vi "PMX-4EX-SA Command Generator.vi"(0 "COMMAND":T1=enum."getDeviceId", 5 "args":string[](array[string]), 7 "AXIS":u16(ring) items=["X", "Y", "Z", "U"]) -> (6 "COMMAND":string)   [LabVIEW 2018]
doc: "converts a user friendly request to an actual (raw) string command for the Performax API\n\nProduced By:\n\nChristopher Lemieux\nTest and Automation Engineer\ntestengnr@yahoo.com"
uses:
  PerformaxLV_v103.llb/commandsnew.ctl
panel:
  # "LIBRARY FILE ADJUSTED FOR X,Y,Z,U"
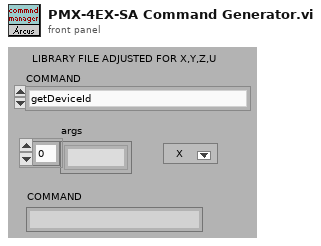
[diagram p1: front panel]
types:
  T1 = typedef "commandsnew.ctl" = enum16{"clearErr", "constJogNeg", "constJogPos", "getAccel", "getDeviceId", "getFirmwareVer", "getHighSpeed", "getIdleAmp", "getLowSpeed", "getMicroStep", "getMotorStatus", "getPolarity", "getPosition", "getProdId", "getPwrStatus", "getRunAmp", "getStatus", "getTemp", "homeNeg", "homePos", "moveToPosition", "powerDown", "powerUp", "setAccel", "setDeviceId", "setHighSpeed", "setIdleAmp", "setLowSpeed", "setMicroStep", "setPolarityLow", "setPolarityHigh", "setPosition", "setRunAmp", "stopFast", "stopSlow"}
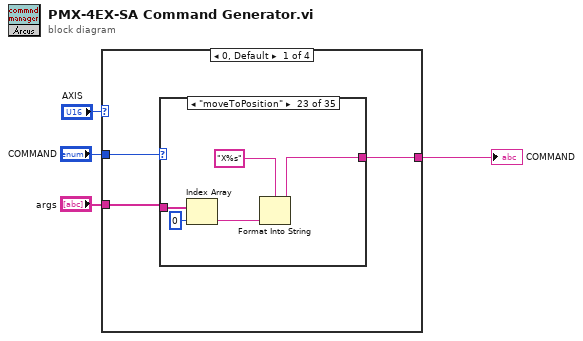
[diagram p0: block diagram]
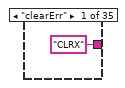
[diagram p2: hidden frame]
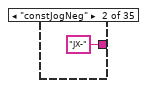
[diagram p3: hidden frame]
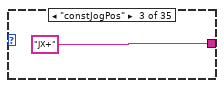
[diagram p4: hidden frame]
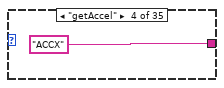
[diagram p5: hidden frame]
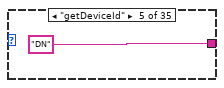
[diagram p6: hidden frame]
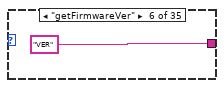
[diagram p7: hidden frame]
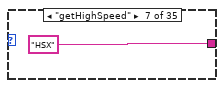
[diagram p8: hidden frame]
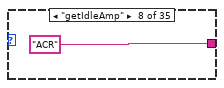
[diagram p9: hidden frame]
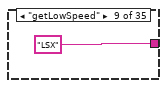
[diagram p10: hidden frame]
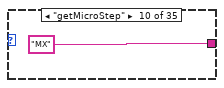
[diagram p11: hidden frame]
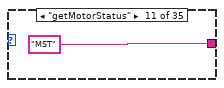
[diagram p12: hidden frame]
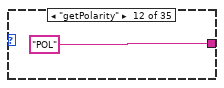
[diagram p13: hidden frame]
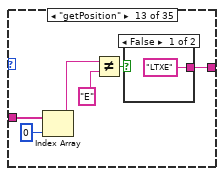
[diagram p14: hidden frame]
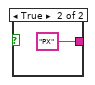
[diagram p15: hidden frame]
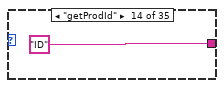
[diagram p16: hidden frame]
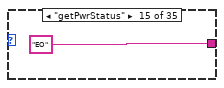
[diagram p17: hidden frame]
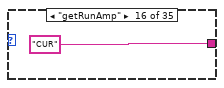
[diagram p18: hidden frame]
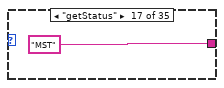
[diagram p19: hidden frame]
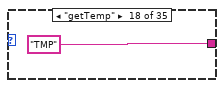
[diagram p20: hidden frame]
diagram:
  n1 = case shown="0, Default" "AXIS" {
    tunnel: "COMMAND" -> [w5 w88 w168 w249]
    tunnel: [w7 w87 w169 w250] -> w1
    tunnel: "args" -> [w6 w86 w167 w248]
    frame 0, Default {
      n2 = case shown="\"moveToPosition\"" w5 {
        tunnel: ["CLRX" "JX-" "JX+" "ACCX" "DN" "VER" "HSX" "ACR" "LSX" "MX" "MST" "POL" w25 "ID" "EO" "CUR" "MST" "TMP" "HX-" "HX+" "EO1=0" "EO1=1" w37 w42 w47 w52 w57 w62 w67 w72 w77 "ABORT" "STOPX" "POL=0" "POL=1"] -> w7
        tunnel: w6 -> [_ _ _ _ _ _ _ _ _ _ _ _ w24 _ _ _ _ _ _ _ _ _ w40 w45 w50 w55 w60 w65 w70 w75 w80 _ _ _ _]
        frame "clearErr" {
        }
        frame "constJogNeg" {
        }
        frame "constJogPos" {
        }
        frame "getAccel" {
        }
        frame "getDeviceId" {
        }
        frame "getFirmwareVer" {
        }
        frame "getHighSpeed" {
        }
        frame "getIdleAmp" {
        }
        frame "getLowSpeed" {
        }
        frame "getMicroStep" {
        }
        frame "getMotorStatus" {
        }
        frame "getPolarity" {
        }
        frame "getPosition" {
          n3 = Index Array(array=w24, index=0) -> (element=w21:string)
          n4 = Not Equal?(x=w21, y="E") -> (x != y?=w22:bool)
          n5 = case shown="False" w22 {
            tunnel: ["LTXE" "PX"] -> w25
            frame False {
            }
            frame True {
            }
          }
        }
        frame "getProdId" {
        }
        frame "getPwrStatus" {
        }
        frame "getRunAmp" {
        }
        frame "getStatus" {
        }
        frame "getTemp" {
        }
        frame "homeNeg" {
        }
        frame "homePos" {
        }
        frame "powerDown" {
        }
        frame "powerUp" {
        }
        frame "moveToPosition" {
          n6 = Index Array(array=w40, index=0) -> (element=w38:string)
          n7 = Format Into String(format string="X%s", w38) -> (resulting string=w37:string)  [unwired: 2 in, 1 out]
        }
        frame "setAccel" {
          n8 = Index Array(array=w45, index=0) -> (element=w43:string)
          n9 = Format Into String(format string="ACCX=%s", w43) -> (resulting string=w42:string)  [unwired: 2 in, 1 out]
        }
        frame "setDeviceId" {
          n10 = Index Array(array=w50, index=0) -> (element=w48:string)
          n11 = Format Into String(format string="DN=%s", w48) -> (resulting string=w47:string)  [unwired: 2 in, 1 out]
        }
        frame "setHighSpeed" {
          n12 = Index Array(array=w55, index=0) -> (element=w53:string)
          n13 = Format Into String(format string="HSX=%s", w53) -> (resulting string=w52:string)  [unwired: 2 in, 1 out]
        }
        frame "setIdleAmp" {
          n14 = Index Array(array=w60, index=0) -> (element=w58:string)
          n15 = Format Into String(format string="ACR=%s", w58) -> (resulting string=w57:string)  [unwired: 2 in, 1 out]
        }
        frame "setLowSpeed" {
          n16 = Index Array(array=w65, index=0) -> (element=w63:string)
          n17 = Format Into String(format string="LSX=%s", w63) -> (resulting string=w62:string)  [unwired: 2 in, 1 out]
        }
        frame "setMicroStep" {
          n18 = Index Array(array=w70, index=0) -> (element=w68:string)
          n19 = Format Into String(format string="MX=%s", w68) -> (resulting string=w67:string)  [unwired: 2 in, 1 out]
        }
        frame "setPosition" {
          n20 = Index Array(array=w75, index=0) -> (element=w73:string)
          n21 = Format Into String(format string="PX=%s", w73) -> (resulting string=w72:string)  [unwired: 2 in, 1 out]
        }
        frame "setRunAmp" {
          n22 = Index Array(array=w80, index=0) -> (element=w78:string)
          n23 = Format Into String(format string="CUR=%s", w78) -> (resulting string=w77:string)  [unwired: 2 in, 1 out]
        }
        frame "stopFast" {
        }
        frame "stopSlow" {
        }
        frame "setPolarityLow" {
        }
        frame "setPolarityHigh" {
        }
      }
    }
    frame 1 {
      n24 = case shown="\"getDeviceId\"" w88 {
        tunnel: ["CLRY" "JY-" "JY+" "ACCY" "DN" "VER" "HSY" "ACR" "LSY" "MX" "MST" "POL" w101 "ID" "EO" "CUR" "MST" "TMP" "HY-" "HY+" "EO2=0" "EO2=1" w118 w123 w128 w133 w138 w143 w148 w153 w158 "ABORT" "STOPY" "POL=0" "POL=1"] -> w87
        tunnel: w86 -> [_ _ _ _ _ _ _ _ _ _ _ _ w102 _ _ _ _ _ _ _ _ _ w121 w126 w131 w136 w141 w146 w151 w156 w161 _ _ _ _]
        frame "clearErr" {
        }
        frame "constJogNeg" {
        }
        frame "constJogPos" {
        }
        frame "getAccel" {
        }
        frame "getDeviceId" {
        }
        frame "getFirmwareVer" {
        }
        frame "getHighSpeed" {
        }
        frame "getIdleAmp" {
        }
        frame "getLowSpeed" {
        }
        frame "getMicroStep" {
        }
        frame "getMotorStatus" {
        }
        frame "getPolarity" {
        }
        frame "getPosition" {
          n25 = Index Array(array=w102, index=0) -> (element=w105:string)
          n26 = Not Equal?(x=w105, y="E") -> (x != y?=w104:bool)
          n27 = case shown="True" w104 {
            tunnel: ["LTYE" "PY"] -> w101
            frame False {
            }
            frame True {
            }
          }
        }
        frame "getProdId" {
        }
        frame "getPwrStatus" {
        }
        frame "getRunAmp" {
        }
        frame "getStatus" {
        }
        frame "getTemp" {
        }
        frame "homeNeg" {
        }
        frame "homePos" {
        }
        frame "powerDown" {
        }
        frame "powerUp" {
        }
        frame "moveToPosition" {
          n28 = Index Array(array=w121, index=0) -> (element=w119:string)
          n29 = Format Into String(format string="Y%s", w119) -> (resulting string=w118:string)  [unwired: 2 in, 1 out]
        }
        frame "setAccel" {
          n30 = Index Array(array=w126, index=0) -> (element=w124:string)
          n31 = Format Into String(format string="ACCY=%s", w124) -> (resulting string=w123:string)  [unwired: 2 in, 1 out]
        }
        frame "setDeviceId" {
          n32 = Index Array(array=w131, index=0) -> (element=w129:string)
          n33 = Format Into String(format string="DN=%s", w129) -> (resulting string=w128:string)  [unwired: 2 in, 1 out]
        }
        frame "setHighSpeed" {
          n34 = Index Array(array=w136, index=0) -> (element=w134:string)
          n35 = Format Into String(format string="HSY=%s", w134) -> (resulting string=w133:string)  [unwired: 2 in, 1 out]
        }
        frame "setIdleAmp" {
          n36 = Index Array(array=w141, index=0) -> (element=w139:string)
          n37 = Format Into String(format string="ACR=%s", w139) -> (resulting string=w138:string)  [unwired: 2 in, 1 out]
        }
        frame "setLowSpeed" {
          n38 = Index Array(array=w146, index=0) -> (element=w144:string)
          n39 = Format Into String(format string="LSY=%s", w144) -> (resulting string=w143:string)  [unwired: 2 in, 1 out]
        }
        frame "setMicroStep" {
          n40 = Index Array(array=w151, index=0) -> (element=w149:string)
          n41 = Format Into String(format string="MX=%s", w149) -> (resulting string=w148:string)  [unwired: 2 in, 1 out]
        }
        frame "setPosition" {
          n42 = Index Array(array=w156, index=0) -> (element=w154:string)
          n43 = Format Into String(format string="PY=%s", w154) -> (resulting string=w153:string)  [unwired: 2 in, 1 out]
        }
        frame "setRunAmp" {
          n44 = Index Array(array=w161, index=0) -> (element=w159:string)
          n45 = Format Into String(format string="CUR=%s", w159) -> (resulting string=w158:string)  [unwired: 2 in, 1 out]
        }
        frame "stopFast" {
        }
        frame "stopSlow" {
        }
        frame "setPolarityLow" {
        }
        frame "setPolarityHigh" {
        }
      }
    }
    frame 2 {
      n46 = case shown="\"getMicroStep\"" w168 {
        tunnel: ["CLRZ" "JZ-" "JZ+" "ACCZ" "DN" "VER" "HSZ" "ACR" "LSZ" "MZ" "MST" "POL" w183 "ID" "EO" "CUR" "MST" "TMP" "HZ-" "HZ+" "EO3=0" "EO3=1" w199 w204 w209 w214 w219 w224 w229 w234 w239 "ABORT" "STOPZ" "POL=0" "POL=1"] -> w169
        tunnel: w167 -> [_ _ _ _ _ _ _ _ _ _ _ _ w182 _ _ _ _ _ _ _ _ _ w202 w207 w212 w217 w222 w227 w232 w237 w242 _ _ _ _]
        frame "clearErr" {
        }
        frame "constJogNeg" {
        }
        frame "constJogPos" {
        }
        frame "getAccel" {
        }
        frame "getDeviceId" {
        }
        frame "getFirmwareVer" {
        }
        frame "getHighSpeed" {
        }
        frame "getIdleAmp" {
        }
        frame "getLowSpeed" {
        }
        frame "getMicroStep" {
        }
        frame "getMotorStatus" {
        }
        frame "getPolarity" {
        }
        frame "getPosition" {
          n47 = Index Array(array=w182, index=0) -> (element=w186:string)
          n48 = Not Equal?(x=w186, y="E") -> (x != y?=w185:bool)
          n49 = case shown="True" w185 {
            tunnel: ["LTZE" "PZ"] -> w183
            frame False {
            }
            frame True {
            }
          }
        }
        frame "getProdId" {
        }
        frame "getPwrStatus" {
        }
        frame "getRunAmp" {
        }
        frame "getStatus" {
        }
        frame "getTemp" {
        }
        frame "homeNeg" {
        }
        frame "homePos" {
        }
        frame "powerDown" {
        }
        frame "powerUp" {
        }
        frame "moveToPosition" {
          n50 = Index Array(array=w202, index=0) -> (element=w200:string)
          n51 = Format Into String(format string="Z%s", w200) -> (resulting string=w199:string)  [unwired: 2 in, 1 out]
        }
        frame "setAccel" {
          n52 = Index Array(array=w207, index=0) -> (element=w205:string)
          n53 = Format Into String(format string="ACCZ=%s", w205) -> (resulting string=w204:string)  [unwired: 2 in, 1 out]
        }
        frame "setDeviceId" {
          n54 = Index Array(array=w212, index=0) -> (element=w210:string)
          n55 = Format Into String(format string="DN=%s", w210) -> (resulting string=w209:string)  [unwired: 2 in, 1 out]
        }
        frame "setHighSpeed" {
          n56 = Index Array(array=w217, index=0) -> (element=w215:string)
          n57 = Format Into String(format string="HSZ=%s", w215) -> (resulting string=w214:string)  [unwired: 2 in, 1 out]
        }
        frame "setIdleAmp" {
          n58 = Index Array(array=w222, index=0) -> (element=w220:string)
          n59 = Format Into String(format string="ACR=%s", w220) -> (resulting string=w219:string)  [unwired: 2 in, 1 out]
        }
        frame "setLowSpeed" {
          n60 = Index Array(array=w227, index=0) -> (element=w225:string)
          n61 = Format Into String(format string="LSZ=%s", w225) -> (resulting string=w224:string)  [unwired: 2 in, 1 out]
        }
        frame "setMicroStep" {
          n62 = Index Array(array=w232, index=0) -> (element=w230:string)
          n63 = Format Into String(format string="MZ=%s", w230) -> (resulting string=w229:string)  [unwired: 2 in, 1 out]
        }
        frame "setPosition" {
          n64 = Index Array(array=w237, index=0) -> (element=w235:string)
          n65 = Format Into String(format string="PZ=%s", w235) -> (resulting string=w234:string)  [unwired: 2 in, 1 out]
        }
        frame "setRunAmp" {
          n66 = Index Array(array=w242, index=0) -> (element=w240:string)
          n67 = Format Into String(format string="CUR=%s", w240) -> (resulting string=w239:string)  [unwired: 2 in, 1 out]
        }
        frame "stopFast" {
        }
        frame "stopSlow" {
        }
        frame "setPolarityLow" {
        }
        frame "setPolarityHigh" {
        }
      }
    }
    frame 3 {
      n68 = case shown="\"homePos\"" w249 {
        tunnel: ["CLRU" "JU-" "JU+" "ACCU" "DN" "VER" "HSU" "ACR" "LSU" "MX" "MST" "POL" w264 "ID" "EO" "CUR" "MST" "TMP" "HU-" "HU+" "EO3=0" "EO4=1" w280 w285 w290 w295 w300 w305 w310 w315 w320 "ABORT" "STOPU" "POL=0" "POL=1"] -> w250
        tunnel: w248 -> [_ _ _ _ _ _ _ _ _ _ _ _ w263 _ _ _ _ _ _ _ _ _ w283 w288 w293 w298 w303 w308 w313 w318 w323 _ _ _ _]
        frame "clearErr" {
        }
        frame "constJogNeg" {
        }
        frame "constJogPos" {
        }
        frame "getAccel" {
        }
        frame "getDeviceId" {
        }
        frame "getFirmwareVer" {
        }
        frame "getHighSpeed" {
        }
        frame "getIdleAmp" {
        }
        frame "getLowSpeed" {
        }
        frame "getMicroStep" {
        }
        frame "getMotorStatus" {
        }
        frame "getPolarity" {
        }
        frame "getPosition" {
          n69 = Index Array(array=w263, index=0) -> (element=w267:string)
          n70 = Not Equal?(x=w267, y="E") -> (x != y?=w266:bool)
          n71 = case shown="False" w266 {
            tunnel: ["LTUE" "PU"] -> w264
            frame False {
            }
            frame True {
            }
          }
        }
        frame "getProdId" {
        }
        frame "getPwrStatus" {
        }
        frame "getRunAmp" {
        }
        frame "getStatus" {
        }
        frame "getTemp" {
        }
        frame "homeNeg" {
        }
        frame "homePos" {
        }
        frame "powerDown" {
        }
        frame "powerUp" {
        }
        frame "moveToPosition" {
          n72 = Index Array(array=w283, index=0) -> (element=w281:string)
          n73 = Format Into String(format string="U%s", w281) -> (resulting string=w280:string)  [unwired: 2 in, 1 out]
        }
        frame "setAccel" {
          n74 = Index Array(array=w288, index=0) -> (element=w286:string)
          n75 = Format Into String(format string="ACCU=%s", w286) -> (resulting string=w285:string)  [unwired: 2 in, 1 out]
        }
        frame "setDeviceId" {
          n76 = Index Array(array=w293, index=0) -> (element=w291:string)
          n77 = Format Into String(format string="DN=%s", w291) -> (resulting string=w290:string)  [unwired: 2 in, 1 out]
        }
        frame "setHighSpeed" {
          n78 = Index Array(array=w298, index=0) -> (element=w296:string)
          n79 = Format Into String(format string="HSU=%s", w296) -> (resulting string=w295:string)  [unwired: 2 in, 1 out]
        }
        frame "setIdleAmp" {
          n80 = Index Array(array=w303, index=0) -> (element=w301:string)
          n81 = Format Into String(format string="ACR=%s", w301) -> (resulting string=w300:string)  [unwired: 2 in, 1 out]
        }
        frame "setLowSpeed" {
          n82 = Index Array(array=w308, index=0) -> (element=w306:string)
          n83 = Format Into String(format string="LSU=%s", w306) -> (resulting string=w305:string)  [unwired: 2 in, 1 out]
        }
        frame "setMicroStep" {
          n84 = Index Array(array=w313, index=0) -> (element=w311:string)
          n85 = Format Into String(format string="MX=%s", w311) -> (resulting string=w310:string)  [unwired: 2 in, 1 out]
        }
        frame "setPosition" {
          n86 = Index Array(array=w318, index=0) -> (element=w316:string)
          n87 = Format Into String(format string="PU=%s", w316) -> (resulting string=w315:string)  [unwired: 2 in, 1 out]
        }
        frame "setRunAmp" {
          n88 = Index Array(array=w323, index=0) -> (element=w321:string)
          n89 = Format Into String(format string="CUR=%s", w321) -> (resulting string=w320:string)  [unwired: 2 in, 1 out]
        }
        frame "stopFast" {
        }
        frame "stopSlow" {
        }
        frame "setPolarityLow" {
        }
        frame "setPolarityHigh" {
        }
      }
    }
  }
  "COMMAND" <- w1
